vi "RealtimeDNITrack_Optimized.vi"() -> ()   [LabVIEW 2017]
uses:
  <extravilib>/ChannelInstances/Tag-bool.lvlib
  <vilib>/platform/TimedLoop/XDataNode/XDataNode.xnode
  <vilib>/Platform/TimedLoop/XDataNode/nitl_modes.ctl
  <vilib>/Platform/TimedLoop/XDataNode/XDNodeRunTimeDep.lvlib
  <vilib>/Platform/TimedLoop/XDataNode/wakeup.ctl
  <vilib>/Platform/TimedLoop/XDataNode/timing_clust.ctl
  <vilib>/daq.io/MQTT LabVIEW Client/MQTT_Functions.lvlib
  <vilib>/daq.io/MQTT LabVIEW Client/Controls/MessageType.ctl
  <vilib>/daq.io/MQTT LabVIEW Client/Controls/Retain_Flag.ctl
  <vilib>/daq.io/MQTT LabVIEW Client/Controls/DUP_Flag.ctl
  <vilib>/daq.io/MQTT LabVIEW Client/Controls/QoS.ctl
  <vilib>/daq.io/MQTT LabVIEW Client/Controls/Connect_Flags.ctl
  <vilib>/daq.io/MQTT LabVIEW Client/Controls/Connection_Return_Codes.ctl
panel:
  out "MQTT Feed":string
  in  "Tab Control":T1(tab)
  out "Corrected Phi":string
  out "Corrected Theta":string
  out "Current Time":string
  out "Corrected DNI":dbl
  in  "Working Directory":path=path "G:/Chad/Tracking Software/Analysis/LabVIEW-Outdoor-Tracking-App"
  out "Time of tracking start":string
  out "Sunset":string
  out "Sunrise":string
  in  "stop":bool
  in  "Stop Reading":bool
  out "standard error 3":string
  out "return code 3":i32
  in  "Script 3":string="solar_system.py"
  out "standard error":string
  out "return code":i32
  in  "error in (no error)":errorcluster
  in  "Sample Frequency (minutes)":string="1"
  out "Seconds to wait\nfor next minute":dbl
  in  "Script":string="cos_correct_v2.py"
  in  "Script 2":string="angle_to_position.py"
  out "standard error 2":string
  out "return code 2":i32
  out "Time":string
  out "Current Y":dbl
  out "Cos Corrected DNI":cluster{dbl[], dbl[]}(graph)
  out "Tracking":cluster{"X Coords":dbl[], "Y Coords":dbl[]}[](graph)
  out "Current X":dbl
  in  "Show full history":bool
  out "Waveform Graph":dbl[][](graph)
  in  "X Length":i32
  in  "Client ID":string="LVSubscribeClient"
  in  "Connect Flags":T2
  out "Granted QoS Levels":T3[](array[typedef])
  in  "Subscription Info Array":cluster{"Topic":string, "QoS":T3}[](array[cluster])=[{"Topic"="testtopic/LVMQTT", "QoS"=enum."At most once"}]
  in  "MQTT Broker":cluster{"address (IP)":string, "port":u16}={"address (IP)"="192.168.15.7", "port"=1883}
  out "Connection Status":T4=enum."Connection refused: Server unavailable"
  out "Messages":T6(array[cluster])
  in  "Ping period (ms)":u32
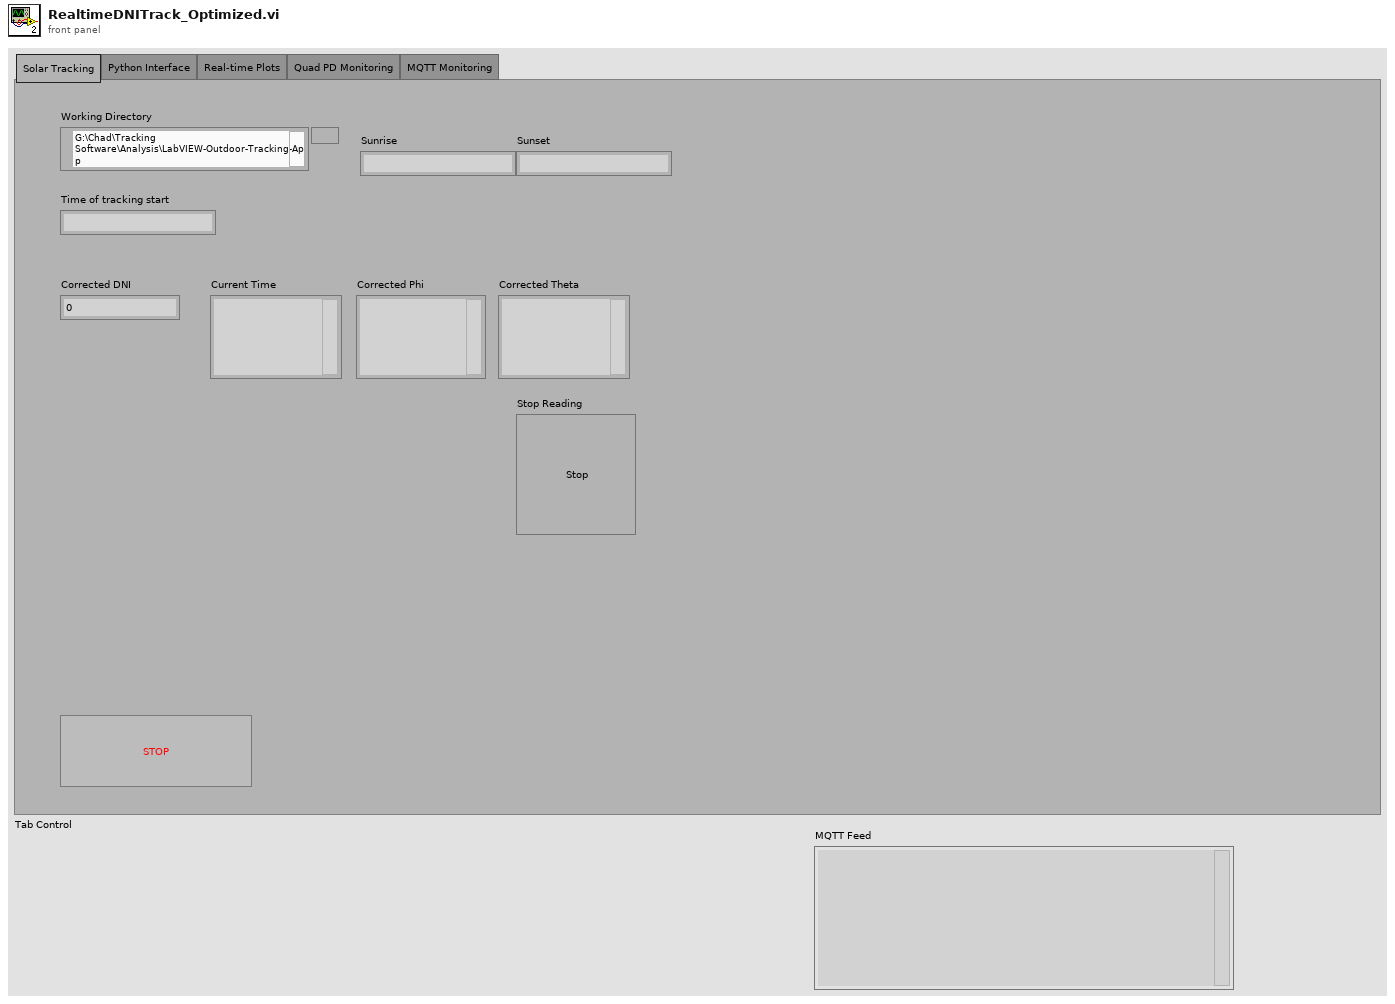
[diagram p1: front panel]
types:
  T1 = enum32{"Solar Tracking", "Python Interface", "Real-time Plots", "Quad PD Monitoring", "MQTT Monitoring"}
  T2 = typedef "MQTT_Functions.lvlib/Connect_Flags.ctl" = cluster{"user name":bool, "password":bool, "will retain":bool, "will flag":bool, "clean session":bool, "reserved":bool, "will QoS":T3}
  T3 = typedef "MQTT_Functions.lvlib/QoS.ctl" = enum8{"At most once", "At least once", "Exactly once", "Reserved"}
  T4 = typedef "MQTT_Functions.lvlib/Connection_Return_Codes.ctl" = enum16{"Connection accepted", "Connection refused: unacceptable protocol version", "Connection refused: identifier rejected", "Connection refused: Server unavailable", "Connection refused: bad user name or password", "Connection refused: not authorized"}
  T5 = typedef "MQTT_Functions.lvlib/MessageType.ctl" = enum32{"Reserved", "CONNECT", "CONNACK", "PUBLISH", "PUBACK", "PUBREC", "PUBREL", "PUBCOMP", "SUBSCRIBE", "SUBACK", "UNSUBSCRIBE", "UNSUBACK", "PINGREQ", "PINGRESP", "DISCONNECT", "Reserved2"}
  T6 = cluster{"Message ID":u16, "Topic Name":string, "Message ":string, "MessageType":T5}[]
  T7 = typedef "XDNodeRunTimeDep.lvlib/timing_clust.ctl" = cluster{"Expected End [f-1]":u64, "Actual End [f-1]":u64, "Finished Late? [f-1]":bool, "Expected End [i-1]":u64, "Actual End [i-1]":u64, "Finished Late? [i-1]":bool, "Expected Start [i]":u64, "Actual Start [i]":u64, "Expected Start [f]":u64, "Actual Start [f]":u64, "Source Name":string, "Structure Name":string, "Period":i64, "Deadline":i64, "Offset":i64, "Start":i64, "Priority":i32, "Timeout":i32, "Mode":T8, "Wakeup Reason":T9, "Error":errorcluster, "Source Type":string, "Secondary Source Type":string, "Global End Time":u64, "Global Start Time":u64, "Frame Duration":u64, "Iteration Duration":u64, "Assigned CPU":i32, "I/O Scan Engine Mode":u32}
  T8 = typedef "XDNodeRunTimeDep.lvlib/nitl_modes.ctl" = enum32{"No Change", "Process missed periods, maintain original phase", "Discard missed periods, maintain original phase", "Process missed periods, ignore original phase", "Discard missed periods, ignore original phase"}
  T9 = typedef "XDNodeRunTimeDep.lvlib/wakeup.ctl" = enum32{"Normal", "Aborted", "Asynchronous wakeup", "Timing source error", "Timed loop error", "Timeout"}
  T10 = typedef "MQTT_Functions.lvlib/DUP_Flag.ctl" = bool
  T11 = typedef "MQTT_Functions.lvlib/Retain_Flag.ctl" = bool
  T12 = cluster{"QoS":T3, "DUP":T10, "Retain":T11, "Keep Alive (sec)":u16}
  T13 = enum16{"None", "On Hover", "On Key Focus", "On Hover or Key Focus"}
  T14 = cluster{"Message ID":u16, "Topic Name":string, "Message":string, "MessageType":T5}[]
  T15 = cluster{"Message ID":u16, "Topic Name":string, "Message":string, "MessageType":T5}
  T16 = cluster{"Value[0]":cluster{"X Coords":dbl[], "Y Coords":dbl[]}, "Value[1]":cluster{"X Coords":dbl[], "Y Coords":dbl[]}, "Value[2]":cluster{"X Coords":dbl[], "Y Coords":dbl[]}, "Value[3]":cluster{"X Coords":dbl[], "Y Coords":dbl[]}, "Value[4]":cluster{"X Coords":dbl[], "Y Coords":dbl[]}, "Value[5]":cluster{"X Coords":dbl[], "Y Coords":dbl[]}, "Value[6]":cluster{"X Coords":dbl[], "Y Coords":dbl[]}, "Value[7]":cluster{"X Coords":dbl[], "Y Coords":dbl[]}, "Value[8]":cluster{"X Coords":dbl[], "Y Coords":dbl[]}}
  T17 = cluster{"Value[0]":cluster{"X Coords":dbl[], "Y Coords":dbl[]}, "Value[1]":cluster{"X Coords":dbl[], "Y Coords":dbl[]}, "Value[2]":cluster{"X Coords":dbl[], "Y Coords":dbl[]}}
  T18 = cluster{cluster{dbl[], dbl[]}, cluster{dbl[], dbl[]}, cluster{dbl[], dbl[]}}
  T19 = cluster{cluster{"X Coords":dbl[], "Y Coords":dbl[]}, cluster{dbl[], dbl[]}, "Value[2]":cluster{"X Coords":dbl[], "Y Coords":dbl[]}}
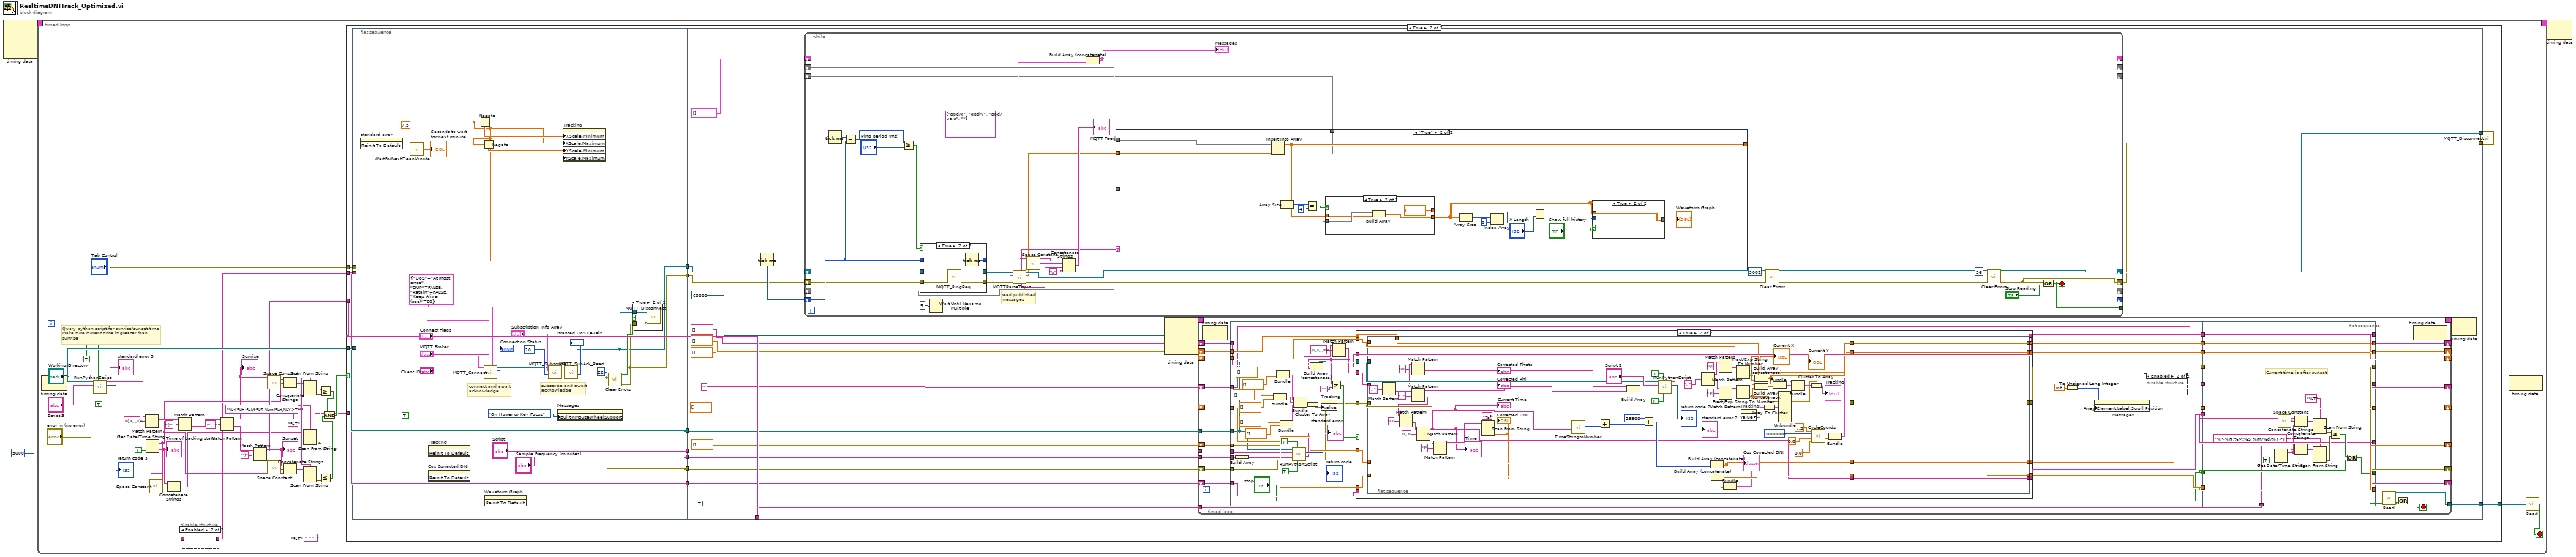
[diagram p0: block diagram]
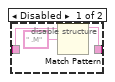
[diagram p2: hidden frame]
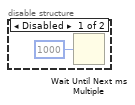
[diagram p5: hidden frame]
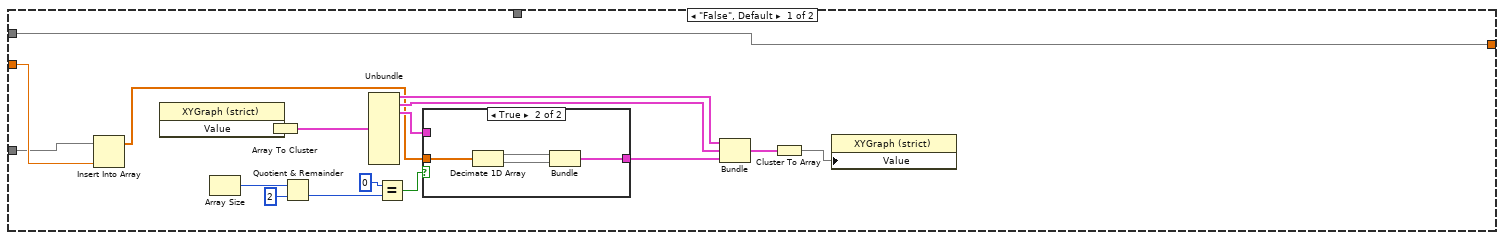
[diagram p7: hidden frame]
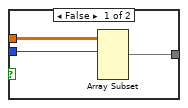
[diagram p9: hidden frame]
diagram:
  n1 = node-c288(i64 5000 ("Period")) -> (w3:T7)  [unwired: 3 in]
  n2 = timed-loop {
    timing: w3 -> [_]
    timing-out: [_] -> w2
    stop <- w41 stop-if-true
    w8 = "%<%H:%M:%S %m/%d/%Y>T" ("format string")
    (unwired) "%T" ("format string")
    (unwired) ".?.:.." ("regular expression")
    # "Query python script for sunrise/sunset time\nMake sure current time is greater than\nsunrise"
    n3 = node-c288() -> ()  [unwired: 1 in, 1 out]
    n4 = call "RunPythonScript.vi"("Run minimized? (F)"=TRUE, "Wait until completion? (T)"=TRUE, "error in (no error)"="error in (no error)", "Script"="Script 3", "Script Directory"="Working Directory") -> ("error out"=w23:errorcluster, "standard error"=→"standard error 3":string, "return code"=→"return code 3":i32, "standard output"=w37:string)  [unwired: 3 in]
    n5 = Match Pattern(string=w37, regular expression="(.*, .*)") -> (match substring=w36:string)  [unwired: 1 in, 3 out]
    n6 = Get Date/Time String(want seconds? (F)=TRUE) -> (date string=w14:string, time string=w5:string)  [unwired: 2 in]
    "Time of tracking start" <- w5
    n7 = call <vilib>:"Space Constant.vi"() -> ("String"=w22:string)
    n8 = Concatenate Strings(w5, w22, w14) -> (w6:string)
    n9 = Match Pattern(string=w36, regular expression="('") -> (after substring=w32:string)  [unwired: 1 in, 3 out]
    n10 = disable-structure shown="Enabled" {
      disable-tunnel: w5 -> [w44 w45]
      disable-tunnel: [w42 w45] -> w4
      frame Disabled {
        n11 = Match Pattern(string=w44, regular expression=" .M") -> (before substring=w42:string)  [unwired: 1 in, 3 out]
      }
      frame Enabled {
      }
    }
    n12 = Match Pattern(string=w32, regular expression="', '") -> (before substring=w19:string, after substring=w31:string)  [unwired: 1 in, 2 out]
    "Sunrise" <- w19
    n13 = Match Pattern(string=w31, regular expression="')") -> (before substring=w15:string)  [unwired: 1 in, 3 out]
    "Sunset" <- w15
    n14 = call <vilib>:"Space Constant.vi"() -> ("String"=w21:string)
    n15 = call <vilib>:"Space Constant.vi"() -> ("String"=w17:string)
    n16 = Concatenate Strings(w19, w21, w14) -> (w20:string)
    n17 = Concatenate Strings(w15, w17, w14) -> (w16:string)
    n18 = Scan From String(format string=w8, input string=w20) -> (output 1=w24:timestamp)  [unwired: 3 in, 3 out]
    n19 = Scan From String(format string="%T", input string=w6) -> (output 1=w18:timestamp)  [unwired: 3 in, 3 out]
    n20 = Scan From String(format string=w8, input string=w16) -> (output 1=w13:timestamp)  [unwired: 3 in, 3 out]
    n21 = Greater Or Equal?(x=w18, y=w24) -> (x >= y?=w12:bool)
    n22 = Less Or Equal?(x=w18, y=w13) -> (x <= y?=w11:bool)
    n23 = And(x=w12, y=w11) -> (x .and. y?=w10:bool)
    n24 = case shown="True" w10 {
      tunnel: "Working Directory" -> [_ w55]
      tunnel: w23 -> [_ w54]
      tunnel: w15 -> [_ w52]
      tunnel: [_ w53] -> w9
      tunnel: w6 -> [_ _]
      tunnel: w4 -> [_ w50]
      frame False {
      }
      frame True {
        n25 = flat-sequence {
          tunnel: [w64] -> w56
          tunnel: ["Script"] -> w57
          tunnel: [w82] -> w58
          tunnel: ["Sample Frequency (minutes)"] -> w59
          tunnel: w55 -> [w82]
          tunnel: w54 -> [w81]
          tunnel: w50 -> [w78]
          tunnel: [w78] -> w51
          tunnel: [w61] -> w49
          tunnel: [w60] -> w46
          tunnel: w59 -> [w104]
          tunnel: w58 -> [w105]
          tunnel: w57 -> [w106]
          tunnel: w56 -> [w100]
          tunnel: [w93] -> w53
          tunnel: w52 -> [w102]
          tunnel: w51 -> [w101]
          tunnel: w49 -> [w96]
          tunnel: [w94] -> w48
          tunnel: [w97] -> w47
          tunnel: w46 -> [w95]
          frame #0 {
            w79 = TRUE ("Vertical Scrollbar Visible")
            w85 = 7.5
            # "connect and await\nacknowledge"
            # "subscribe and await\nacknowledge"
            n26 = invoke on="standard error" class="Str" method="Reinit To Default"() -> ()  [unwired: 3 in, 3 out]
            n27 = call "WaitForNextCleanMinute.vi"() -> ("Seconds to wait"=→"Seconds to wait\nfor next minute":dbl)  [unwired: 1 in]
            n28 = invoke on="Tracking" class="XYGraph (strict)" method="Reinit To Default"() -> ()  [unwired: 3 in, 3 out]
            n29 = invoke on="Cos Corrected DNI" class="XYGraph (strict)" method="Reinit To Default"() -> ()  [unwired: 3 in, 3 out]
            n30 = Negate(x=w85) -> (-x=w87:dbl)
            n31 = Negate(x=w85) -> (-x=w86:dbl)
            n32 = call <vilib>:"MQTT_Connect.vi"("Connect Meta"=T12 {"QoS"=enum."At most once", "DUP"=FALSE, "Retain"=FALSE, "Keep Alive (sec)"=60}, "Client ID"="Client ID", "Connect Flags"="Connect Flags", "error in (no error)"=w81, "MQTT Broker"="MQTT Broker") -> ("error out"=w66:errorcluster, "Connection Status"=→"Connection Status":T4, "connection ID out"=w68:refnum<k5>)  [unwired: 4 in]
            n33 = invoke on="Waveform Graph" class="WFGraph (strict)" method="Reinit To Default"() -> ()  [unwired: 3 in, 3 out]
            n34 = call <vilib>:"MQTT_Subscribe.vi"("error in (no error)"=w66, "Message ID"=u16 20, "Subscription Info Array"="Subscription Info Array", "connection ID"=w68) -> ("error out"=w72:errorcluster, "connection ID out"=w73:refnum<k5>)  [unwired: 6 in]
            n35 = property on="Messages" class="Arr (strict)"("BuiltInMouseWheelSupport"=T13."On Hover or Key Focus" ("Built-In Mouse Wheel Support")) -> ()  [unwired: 2 in, 2 out]
            n36 = property on="Tracking" class="XYGraph (strict)"("XScale.Minimum"=w87, "XScale.Maximum"=w85, "YScale.Minimum"=w86, "YScale.Maximum"=w85) -> ()  [unwired: 2 in, 2 out]
            n37 = call <vilib>:"MQTT_SubAck_Read.vi"("error in (no error)"=w72, "connection ID"=w73) -> ("error out"=w64:errorcluster, "Granted QoS Levels"=→"Granted QoS Levels":T3[], "connection ID out"=w60:refnum<k5>)  [unwired: 7 in]
            n38 = call <vilib>:"Clear Errors.vi"("error in (no error)"=w64, "specific error code to clear (0: all)"=66) -> ("error out"=w61:errorcluster, "specific error cleared?"=w62:bool)  [unwired: 4 in]
            n39 = case shown="True" w62 {
              tunnel: w60 -> [_ w89]
              tunnel: w61 -> [_ w88]
              frame False {
              }
              frame True {
                n40 = call <vilib>:"MQTT_Disconnect.vi"("error in (no error)"=w88, "connection ID"=w89) -> ()  [unwired: 9 in, 1 out]
              }
            }
          }
          frame #1 {
            (unwired) TRUE ("Key Focus")
            n41 = Tick Count (ms)() -> (millisecond timer value=w98:u32)
            n42 = while {
              shift-right: [w328] -> _
              shift-left: T14 [] ("Array") -> [w336]
              shift-right: [w332] -> w94
              shift-left: w96 -> [w338]
              shift-right: [w320] -> w97
              shift-left: w95 -> [w339]
              shift-right: _ -> [_]
              shift-left: w98 -> [w340]
              shift-right: _ -> [w330]
              shift-left: _ -> [w331]
              shift-right: _ -> [_]
              shift-left: _ -> [w314]
              tunnel: [w329] -> _
              shift-right: _ -> [_]
              shift-left: _ -> [w315]
              stop <- w329 stop-if-true
              # "read published\nmessages"
              n43 = Tick Count (ms)() -> (millisecond timer value=w343:u32)
              n44 = Subtract(x=w343, y=w340) -> (x-y=w341:u32)
              n45 = Greater Or Equal?(x=w341, y="Ping period (ms)") -> (x >= y?=w342:bool)
              n46 = case shown="True" w342 {
                tunnel: [w396 w401] -> _
                tunnel: w340 -> [w396 _]
                tunnel: w338 -> [w394 w400]
                tunnel: w339 -> [w395 w399]
                tunnel: [w394 w398] -> w322
                tunnel: [w395 w397] -> w324
                frame False {
                }
                frame True {
                  n47 = call <vilib>:"MQTT_PingReq.vi"("error in (no error)"=w400, "connection ID"=w399) -> ("error out"=w398:errorcluster, "connection ID out"=w397:refnum<k5>)  [unwired: 7 in, 1 out]
                  n48 = Tick Count (ms)() -> (millisecond timer value=w401:u32)
                }
              }
              n49 = Wait Until Next ms Multiple(millisecond multiple=u32 5) -> ()  [unwired: 1 out]
              n50 = call "MQTTParseTopic.vi"("error in (no error)"=w322, "Array"=string[] ["qpd/x", "qpd/y", "qpd/vals", ""], "connection ID"=w324) -> ("error out"=w321:errorcluster, "Double"=w316:dbl, "connection ID out"=w320:refnum<k5>, "Message"=w319:string, "Topic Name"=w318:string, "output cluster"=w317:T15)  [unwired: 2 in, 1 out]
              n51 = call <vilib>:"Space Constant.vi"() -> ("String"=w327:string)
              n52 = Concatenate Strings(w318, w327, w319, "\r") -> (→"MQTT Feed":string)
              n53 = Build Array (concatenate)(w336, w317) -> (w328:T14)
              "Messages" <- w328
              n54 = case shown="\"True\"" w318 {
                tunnel: w316 -> [w348 w383]
                tunnel: [w362 w369] -> _
                tunnel: w331 -> [w362 w382]
                tunnel: w315 -> [w347 _]
                tunnel: w314 -> [_ w368]
                frame "False", Default {
                  n55 = Insert Into Array(array=w347, new element=w348) -> (w346:dbl[])  [unwired: 1 in]
                  n56 = property on="Property Node" class="XYGraph (strict)"() -> ("Value"=w349:cluster{"X Coords":dbl[], "Y Coords":dbl[]}[])  [unwired: 2 in, 2 out]
                  n57 = Array Size() -> (size(s)=w355:i32)  [unwired: 1 in]
                  n58 = Array To Cluster(array=w349) -> (cluster=w350:T16)
                  n59 = Quotient & Remainder(x=w355, y=2) -> (floor(x/y)=w357:i32)  [unwired: 1 out]
                  n60 = Unbundle(w350) -> ("Value[0]"=w352:cluster{"X Coords":dbl[], "Y Coords":dbl[]}, "Value[1]"=w351:cluster{"X Coords":dbl[], "Y Coords":dbl[]}, "Value[2]"=w361:cluster{"X Coords":dbl[], "Y Coords":dbl[]})  [unwired: 6 out]
                  n61 = Equal?(x=0, y=w357) -> (x = y?=w359:bool)
                  n62 = case shown="True" w359 {
                    tunnel: w346 -> [_ w367]
                    tunnel: [w363 w364] -> w360
                    tunnel: w361 -> [w363 _]
                    frame False {
                    }
                    frame True {
                      n63 = Decimate 1D Array(w367) -> (w366:dbl[], w365:dbl[])
                      n64 = Bundle(w366, w365) -> (w364:cluster{dbl[], dbl[]})  [unwired: 1 in]
                    }
                  }
                  n65 = Bundle("Value[0]"=w352, "Value[1]"=w351, "Value[2]"=w360) -> (w353:T17)  [unwired: 1 in]
                  n66 = Cluster To Array(cluster=w353) -> (array=w354:cluster{"X Coords":dbl[], "Y Coords":dbl[]}[])
                  n67 = property on="Property Node" class="XYGraph (strict)"("Value"=w354) -> ()  [unwired: 2 in, 2 out]
                }
                frame "True" {
                  n68 = Insert Into Array(array=w382, new element=w383) -> (w369:dbl[])  [unwired: 1 in]
                  n69 = Array Size(array=w369) -> (size(s)=w371:i32)
                  n70 = Equal?(x=w371, y=4) -> (x = y?=w372:bool)
                  n71 = case shown="True" w372 {
                    tunnel: w369 -> [w389 w390]
                    tunnel: [w389 dbl[] []] -> w373
                    tunnel: [w388 w392] -> w375
                    tunnel: w368 -> [w388 w391]
                    frame False {
                    }
                    frame True {
                      n72 = Build Array(w391, w390) -> (w392:dbl[][])
                    }
                  }
                  n73 = Array Size(array=w375) -> (size(s)=w377:i32[])
                  n74 = Index Array(array=w377, index=0) -> (element=w379:i32)
                  n75 = Subtract(x=w379, y="X Length") -> (x-y=w380:i32)
                  n76 = case shown="True" "Show full history" {
                    tunnel: [w386 w387] -> w374
                    tunnel: w375 -> [w385 w387]
                    tunnel: w380 -> [w384 _]
                    frame False {
                      n77 = Array Subset(array=w385, index (row)=w384) -> (w386:dbl[][])  [unwired: 3 in]
                    }
                    frame True {
                    }
                  }
                  "Waveform Graph" <- w374
                }
              }
              n78 = call <vilib>:"Clear Errors.vi"("error in (no error)"=w321, "specific error code to clear (0: all)"=5001) -> ("error out"=w333:errorcluster)  [unwired: 4 in, 1 out]
              n79 = call <vilib>:"Clear Errors.vi"("error in (no error)"=w333, "specific error code to clear (0: all)"=56) -> ("error out"=w332:errorcluster)  [unwired: 4 in, 1 out]
              n80 = Or(x=w332, y="Stop Reading") -> (x .or. y?=w329:bool)
            }
            n81 = node-c288(i64 60000 ("Period")) -> (w92:T7)  [unwired: 3 in]
            n82 = timed-loop {
              tunnel: w104 -> [w139]
              shift-right: [w143] -> _
              shift-left: dbl[] [] -> [w144]
              shift-right: [w142] -> _
              shift-left: dbl[] [] -> [w140]
              shift-right: [w132] -> _
              shift-left: string[] [] -> [w141]
              tunnel: w105 -> [w133]
              tunnel: w106 -> [w138]
              shift-right: [w136] -> _
              shift-left: dbl[] [] -> [w135]
              shift-right: [w134] -> _
              shift-left: dbl[] [] -> [w137]
              shift-right: [w124] -> _
              shift-left: w101 -> [w123]
              tunnel: w102 -> [w122]
              tunnel: [w115] -> w93
              shift-right: [w119] -> _
              shift-left: "" -> [w118]
              shift-right: [w121] -> _
              shift-left: w100 -> [w117]
              timing: w92 -> [_]
              timing-out: [_] -> w91
              stop <- w112 stop-if-true
              n83 = node-c288() -> ()  [unwired: 1 in, 1 out]
              n84 = flat-sequence {
                tunnel: w144 -> [w189]
                tunnel: w141 -> [w186]
                tunnel: w140 -> [w185]
                tunnel: w117 -> [w184]
                tunnel: w139 -> [w179]
                tunnel: w138 -> [w177]
                tunnel: w137 -> [w176]
                tunnel: w135 -> [w174]
                tunnel: w133 -> [w172]
                tunnel: [w188] -> w131
                tunnel: [w187] -> w130
                tunnel: [w175] -> w129
                tunnel: ["stop"] -> w128
                tunnel: [w173] -> w127
                tunnel: [w159] -> w126
                tunnel: [w166] -> w125
                tunnel: w123 -> [w165]
                tunnel: [w160] -> w120
                tunnel: w118 -> [w158]
                tunnel: [w158] -> w116
                tunnel: [w305] -> w132
                tunnel: [w306] -> w134
                tunnel: [w307] -> w136
                tunnel: [w308] -> w142
                tunnel: [w309] -> w143
                tunnel: w131 -> [w309]
                tunnel: w130 -> [w308]
                tunnel: w129 -> [w307]
                tunnel: w128 -> [w304]
                tunnel: w127 -> [w306]
                tunnel: w126 -> [w305]
                tunnel: w125 -> [w299]
                tunnel: [w299] -> w124
                tunnel: w122 -> [w297]
                tunnel: [w292] -> w114
                tunnel: [w291] -> w121
                tunnel: w120 -> [w291]
                tunnel: [w290] -> w119
                tunnel: w116 -> [w290]
                frame #0 {
                  n85 = Build Array(w179) -> (w178:string[])
                  n86 = Bundle(dbl[] [], dbl[] []) -> (w149:cluster{dbl[], dbl[]})  [unwired: 1 in]
                  n87 = Bundle(dbl[] [], dbl[] []) -> (w150:cluster{dbl[], dbl[]})  [unwired: 1 in]
                  n88 = Bundle(dbl[] [], dbl[] []) -> (w148:cluster{dbl[], dbl[]})  [unwired: 1 in]
                  n89 = call "RunPythonScript.vi"("Run minimized? (F)"=TRUE ("run minimized? (F)"), "Wait until completion? (T)"=TRUE ("wait until completion? (T)"), "error in (no error)"=w184, "Array of arguments to script"=w178, "Script"=w177, "Script Directory"=w172) -> ("error out"=w161:errorcluster, "standard error"=→"standard error":string, "return code"=→"return code":i32, "standard output"=w181:string)  [unwired: 2 in]
                  n90 = Bundle(w150, w149, w148) -> (w151:T18)  [unwired: 1 in]
                  n91 = Cluster To Array(cluster=w151) -> (array=w147:cluster{dbl[], dbl[]}[])
                  n92 = property on="Tracking" class="XYGraph (strict)"("Value"=w147) -> ()  [unwired: 2 in, 2 out]
                  n93 = Match Pattern(string=w181, regular expression="(.*, .*)") -> (match substring=w169:string)  [unwired: 1 in, 3 out]
                  n94 = Build Array (concatenate)(w186, w169) -> (w167:string[])
                  n95 = Not Equal?(x=w169, y="") -> (x != y?=w168:bool)
                  n96 = case shown="True" w168 {
                    tunnel: w189 -> [w195 w218]
                    tunnel: [w195 w217] -> w188
                    tunnel: [w196 w216] -> w187
                    tunnel: w185 -> [w196 w215]
                    tunnel: w176 -> [w198 w214]
                    tunnel: [w197 w213] -> w175
                    tunnel: w174 -> [w197 w212]
                    tunnel: [w198 w211] -> w173
                    tunnel: w172 -> [_ w210]
                    tunnel: w169 -> [_ w207]
                    tunnel: [w194 w199] -> w159
                    tunnel: w167 -> [w194 w199]
                    tunnel: [w193 w206] -> w166
                    tunnel: w165 -> [w193 _]
                    tunnel: w161 -> [w192 w209]
                    tunnel: [w192 w208] -> w160
                    frame False {
                    }
                    frame True {
                      n97 = flat-sequence {
                        tunnel: w218 -> [w282]
                        tunnel: w215 -> [w274]
                        tunnel: w214 -> [w261]
                        tunnel: w212 -> [w257]
                        tunnel: w210 -> [w244]
                        tunnel: w209 -> [w241]
                        tunnel: w207 -> [w232]
                        tunnel: [w281] -> w205
                        tunnel: [w280] -> w204
                        tunnel: [w260] -> w203
                        tunnel: [w252] -> w202
                        tunnel: [w240] -> w201
                        tunnel: [w222] -> w200
                        tunnel: [w283] -> w206
                        tunnel: [w284] -> w208
                        tunnel: [w285] -> w211
                        tunnel: [w286] -> w213
                        tunnel: [w287] -> w216
                        tunnel: [w288] -> w217
                        tunnel: w205 -> [w288]
                        tunnel: w204 -> [w287]
                        tunnel: w203 -> [w286]
                        tunnel: w202 -> [w285]
                        tunnel: w201 -> [w284]
                        tunnel: w200 -> [w283]
                        frame #0 {
                          n98 = Match Pattern(string=w232, regular expression=", ") -> (before substring=w235:string, after substring=w236:string)  [unwired: 1 in, 2 out]
                          n99 = Match Pattern(string=w235, regular expression="(") -> (after substring=w230:string)  [unwired: 1 in, 3 out]
                          "Corrected Theta" <- w230
                          n100 = Match Pattern(string=w236, regular expression=", ") -> (before substring=w229:string, after substring=w226:string)  [unwired: 1 in, 2 out]
                          "Corrected Phi" <- w229
                          n101 = Match Pattern(string=w226, regular expression="'") -> (after substring=w224:string)  [unwired: 1 in, 3 out]
                          n102 = Match Pattern(string=w224, regular expression="', ") -> (before substring=w222:string, after substring=w223:string)  [unwired: 1 in, 2 out]
                          "Current Time" <- w222
                          "Time" <- w222
                          n103 = Match Pattern(string=w223, regular expression=")") -> (before substring=w228:string)  [unwired: 1 in, 3 out]
                          n104 = Scan From String(format string="%f", input string=w228) -> (output 1=w238:dbl)  [unwired: 3 in, 3 out]
                          "Corrected DNI" <- w238
                          n105 = call "TimeStringtoNumber.vi"("time string"=w222) -> ("Minutes"=w278:i32, "Hours"=w279:i32)  [unwired: 3 out]
                          n106 = Add(x=w279, y=w278) -> (x+y=w277:i32)
                          n107 = Build Array(w230, w229) -> (w271:string[])
                          n108 = Add(x=28800, y=w277) -> (x+y=w275:i32)
                          n109 = call "RunPythonScript.vi"("Run minimized? (F)"=TRUE ("run minimized? (F)"), "Wait until completion? (T)"=TRUE ("wait until completion? (T)"), "error in (no error)"=w241, "Array of arguments to script"=w271, "Script"="Script 2", "Script Directory"=w244) -> ("error out"=w240:errorcluster, "standard error"=→"standard error 2":string, "return code"=→"return code 2":i32, "standard output"=w269:string)  [unwired: 2 in]
                          n110 = Match Pattern(string=w269, regular expression=", ") -> (before substring=w266:string, after substring=w267:string)  [unwired: 1 in, 2 out]
                          n111 = Build Array (concatenate)(w274, w275) -> (w280:dbl[])
                          n112 = Build Array (concatenate)(w282, w238) -> (w281:dbl[])
                          n113 = Match Pattern(string=w266, regular expression="(") -> (after substring=w263:string)  [unwired: 1 in, 3 out]
                          n114 = Match Pattern(string=w267, regular expression=")") -> (before substring=w262:string)  [unwired: 1 in, 3 out]
                          n115 = Bundle(w280, w281) -> (→"Cos Corrected DNI":cluster{dbl[], dbl[]})  [unwired: 1 in]
                          n116 = Fract/Exp String To Number(string=w263) -> (number=w246:dbl)  [unwired: 3 in, 1 out]
                          "Current X" <- w246
                          n117 = Fract/Exp String To Number(string=w262) -> (number=w245:dbl)  [unwired: 3 in, 1 out]
                          "Current Y" <- w245
                          n118 = property on="Tracking" class="XYGraph (strict)"() -> ("Value"=w220:cluster{"X Coords":dbl[], "Y Coords":dbl[]}[])  [unwired: 2 in, 2 out]
                          n119 = Build Array (concatenate)(w257, w246) -> (w260:dbl[])
                          n120 = Build Array (concatenate)(w261, w245) -> (w252:dbl[])
                          n121 = Array To Cluster(array=w220) -> (cluster=w221:T16)
                          n122 = Bundle(w260, w252) -> (w247:cluster{dbl[], dbl[]})  [unwired: 1 in]
                          n123 = Unbundle(w221) -> ("Value[2]"=w219:cluster{"X Coords":dbl[], "Y Coords":dbl[]})  [unwired: 8 out]
                          n124 = call "CircleCoords.vi"("Magnitude"=7.5, "Number of Points"=1000000, "X Origin"=0.0, "Y Origin"=0.0) -> ("X Coords"=w251:dbl[], "Y Coords"=w250:dbl[])  [unwired: 1 in]
                          n125 = Bundle("X Coords"=w251, "Y Coords"=w250) -> (w248:cluster{"X Coords":dbl[], "Y Coords":dbl[]})  [unwired: 1 in]
                          n126 = Bundle(w248, w247, "Value[2]"=w219) -> (w249:T19)  [unwired: 1 in]
                          n127 = Cluster To Array(cluster=w249) -> (array=→"Tracking":cluster{"X Coords":dbl[], "Y Coords":dbl[]}[])
                        }
                        frame #1 {
                        }
                      }
                    }
                  }
                  n128 = To Unsigned Long Integer(number=inf) -> (unsigned 32bit integer=w163:u32)
                  n129 = property on="Messages" class="Arr (strict)"("Array Element.Label.Scroll Position"=w163) -> ()  [unwired: 2 in, 2 out]
                  n130 = disable-structure shown="Enabled" {
                    frame Disabled {
                      n131 = Wait Until Next ms Multiple(millisecond multiple=u32 1000) -> ()  [unwired: 1 out]
                    }
                    frame Enabled {
                    }
                  }
                }
                frame #1 {
                  # "Current time is after sunset"
                  n132 = Get Date/Time String(want seconds? (F)=TRUE) -> (date string=w298:string)  [unwired: 2 in, 1 out]
                  n133 = call <vilib>:"Space Constant.vi"() -> ("String"=w296:string)
                  n134 = Concatenate Strings(w299, w296, w298) -> (w295:string)
                  n135 = Concatenate Strings(w297, w296, w298) -> (w294:string)
                  n136 = Scan From String(format string="%T", input string=w295) -> (output 1=w302:timestamp)  [unwired: 3 in, 3 out]
                  n137 = Scan From String(format string="%<%H:%M:%S %m/%d/%Y>T", input string=w294) -> (output 1=w301:timestamp)  [unwired: 3 in, 3 out]
                  n138 = Greater Or Equal?(x=w302, y=w301) -> (x >= y?=w303:bool)
                  n139 = Or(x=w303, y=w304) -> (x .or. y?=w292:bool)
                }
              }
              n140 = call <extravilib>:"Read.vi"("channel"=w115) -> ("element"=w113:bool)  [unwired: 1 in, 1 out]
              n141 = Or(x=w113, y=w114) -> (x .or. y?=w112:bool)
              n142 = node-c288() -> ()  [unwired: 1 in, 1 out]
            }
            n143 = node-c288(w91) -> ()  [unwired: 1 out]
          }
        }
        n144 = call <vilib>:"MQTT_Disconnect.vi"("error in (no error)"=w48, "connection ID"=w47) -> ()  [unwired: 9 in, 1 out]
      }
    }
    n145 = node-c288() -> ()  [unwired: 1 in, 1 out]
    n146 = call <extravilib>:"Read.vi"("channel"=w9) -> ("element"=w41:bool)  [unwired: 1 in, 1 out]
  }
  n147 = node-c288(w2) -> ()  [unwired: 1 out]
